vi "Read Type.vi"(8 "error in (no error)":errorcluster, 11 "IPS120 in":refnum<class "IPS120.lvclass">) -> (0 "error out":errorcluster, 2 "Type":T1=enum."IPS120", 3 "IPS120 out":refnum<class "IPS120.lvclass">)   [LabVIEW 2015, in "IPS120.lvclass"]
uses:
  IPS120.lvclass
  OO Devices/Device/Device type.ctl
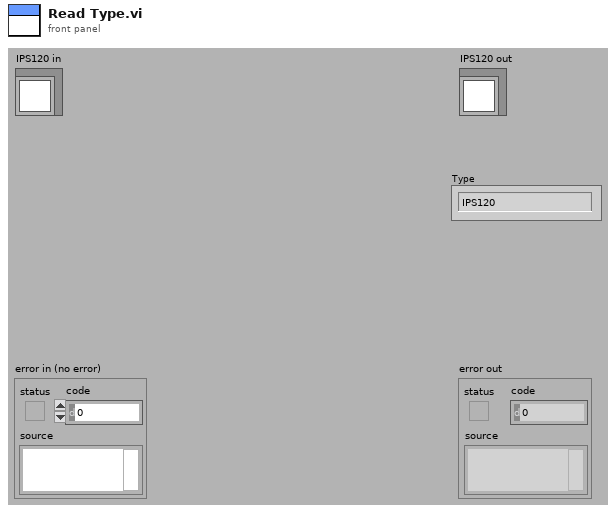
[diagram p1: front panel]
types:
  T1 = typedef "Device type.ctl" = enum16{"NONE", "Neocera 21", "LakeShore 335", "LakeShore 340", "LkShr 340 chA&B", "LakeShore 370", "SRS 850", "SRS 830", "LR 700", "EG&G 5302", "EG&G 7260", "EG&G 7280", "AH 2500", "Keithley meter", "Keithley electrometer", "Keithley 182", "HP 5385", "HP 53181", "HP 53132", "ITC503", "IPS120", "Oxford Mercury IPS", "Oxford PS", "Test", "DC Facility Magnet", "Cryomagnetics PS", "Keithley 2400", "Keithley current source", "Cryo-Con 22C", "HP87NN", "HP4395A"}
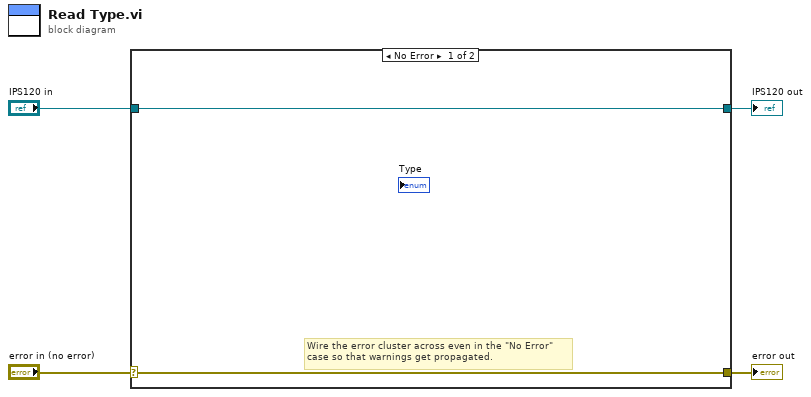
[diagram p0: block diagram]
diagram:
  n1 = case shown="No Error" "error in (no error)" {
    selector: "error in (no error)" -> [w5 w8]
    tunnel: [w5 w8] -> w3
    tunnel: [w6 w7] -> w1
    tunnel: "IPS120 in" -> [w6 w7]
    frame No Error {
      # "Wire the error cluster across even in the \"No Error\"\ncase so that warnings get propagated."
    }
    frame Error {
    }
  }
  "error out" <- w3
  "IPS120 out" <- w1
